vi "COMM prepare data for sending.vi"(11 "data in":variant) -> (3 "data out":variant)   [LabVIEW 2019, in "Communication Interface.lvlib"]
uses:
  Communication Interface.lvlib
  SubVIs/mmWave data_class/mmWave data.lvclass
  <vilib>/Utility/Data Type/NI_Data Type.lvlib
panel:
  out "qualified LabVIEW class name":string[](array[string])
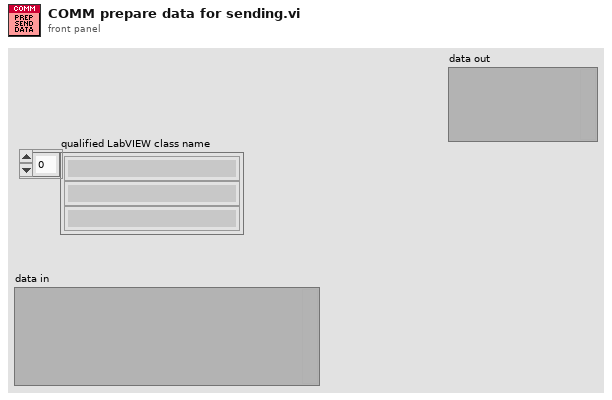
[diagram p1: front panel]
types:
  T1 = typedef "NI_Data Type.lvlib/Data Type.ctl" = enum8{"Invalid Type", "Void", "I8", "I16", "I32", "I64", "U8", "U16", "U32", "U64", "Single Float", "Double Float", "Extended Float", "Single Complex", "Double Complex", "Extended Complex", "Enum U8", "Enum U16", "Enum U32", "Enum U64", "Single Float With Unit", "Double Float With Unit", "Extended Float With Unit", "Single Complex with Unit", "Double Complex with Unit", "Extended Complex with Unit", "Boolean", "String", "Path", "Picture", "Tag", "Array", "Cluster", "Variant", "LV Variant", "Waveform", "Timestamp", "Digital Waveform", "Digital Data", "ExpressData", "Refnum", "External Data", "VI", "Poly VI", "LabVIEW Class Instance", "Fixed Point", "Set Collection", "Map Collection"}
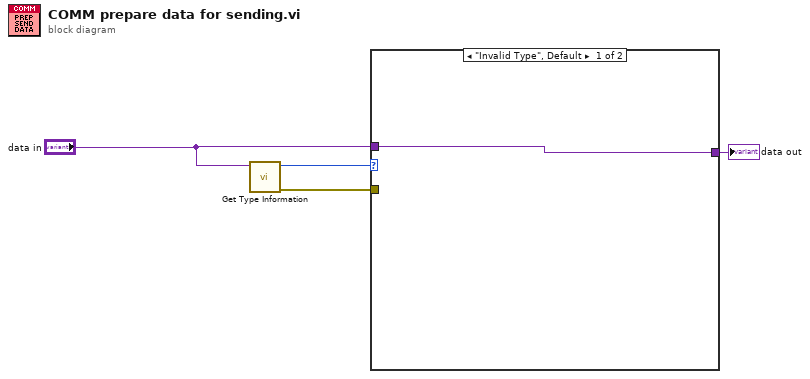
[diagram p0: block diagram]
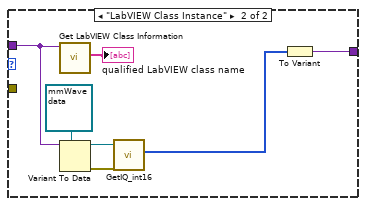
[diagram p2: hidden frame]
diagram:
  n1 = call <vilib>:"Get Type Information.vi"("variant"="data in") -> ("error out"=w4:errorcluster, "type"=w3:T1)  [unwired: 6 in, 3 out]
  n2 = case shown="\"Invalid Type\", Default" w3 {
    tunnel: w4 -> [_ _]
    tunnel: "data in" -> [w5 w11]
    tunnel: [w5 w6] -> w1
    frame "Invalid Type", Default {
    }
    frame "LabVIEW Class Instance" {
      n3 = call <vilib>:"Get LabVIEW Class Information.vi"("variant"=w11) -> ("qualified LabVIEW class name"=→"qualified LabVIEW class name":string[])  [unwired: 8 in, 2 out]
      n4 = Variant To Data(type=refnum<class "mmWave data.lvclass"> refnum ("mmWave data"), Variant=w11) -> (data=w8:refnum<class "mmWave data.lvclass">, error out=w9:errorcluster)  [unwired: 1 in]
      n5 = call-dynamic "GetIQ_int16.vi"("error in (no error)"=w9, "reference in"=w8) -> ("data"=w7:i16[])  [unwired: 6 in, 3 out]
      n6 = To Variant(anything=w7) -> (Variant=w6:variant)
    }
  }
  "data out" <- w1
